vi "Test Parse State from Frame Name.vi"(8 "error in (no error)":errorcluster) -> (0 "error out":errorcluster)   [LabVIEW 2013, in "TEST JKI State Machine API.lvlib"]
uses:
  TEST JKI State Machine API.lvlib
  <vilib>/addons/_JKI Toolkits/Caraya/classes/Assert/Assert.lvclass
  <vilib>/addons/_JKI Toolkits/Caraya/classes/Test/Test.lvclass
  source/JKI SM/JKI SM.lvclass
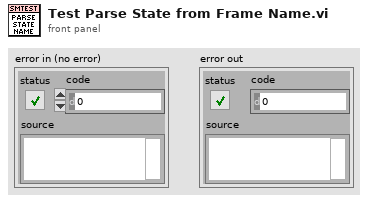
[diagram p1: front panel]
types:
  T1 = cluster{"Frame Name":string, "Exp'd Category":string, "Exp'd State":string, "Comment":string}[]
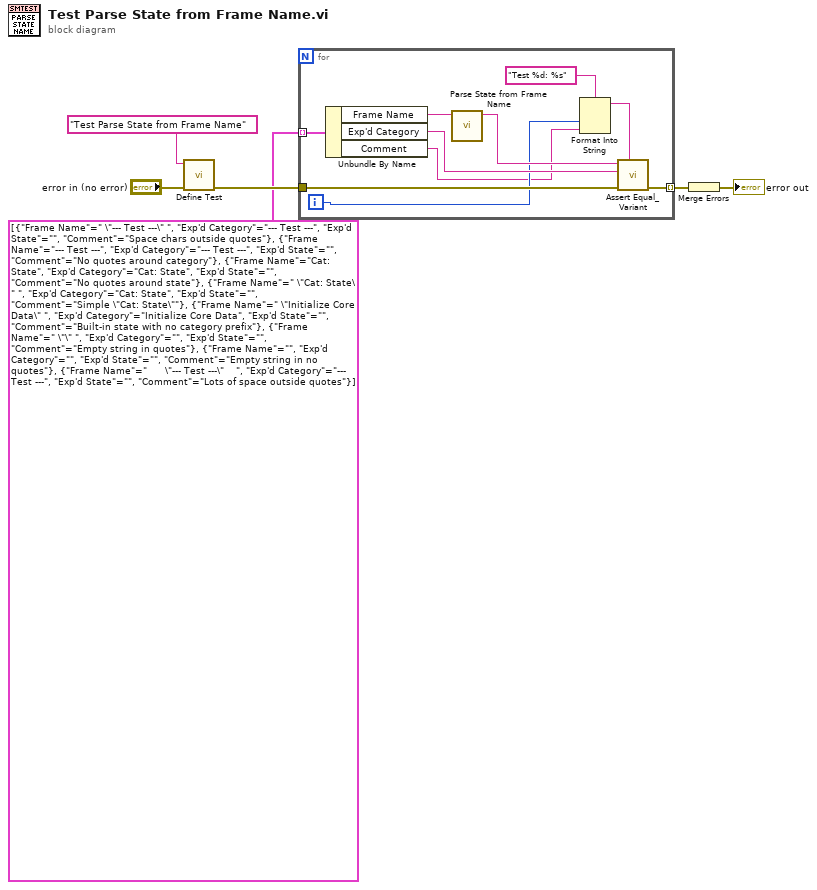
[diagram p0: block diagram]
diagram:
  n1 = call <vilib>:"Define Test.vi"("error in (no error)"="error in (no error)", "Label (VI Title)"="Test Parse State from Frame Name") -> ("error out"=w3:errorcluster)  [unwired: 9 in]
  n2 = for {
    tunnel: [w16] -> w4 mode=indexing
    tunnel: w3 -> [w15]
    tunnel: T1 [{"Frame Name"=" \"--- Test ---\" ", "Exp'd Category"="--- Test ---", "Exp'd State"="", "Comment"="Space chars outside quotes"}, {"Frame Name"="--- Test ---", "Exp'd Category"="--- Test ---", "Exp'd State"="", "Comment"="No quotes around category"}, {"Frame Name"="Cat: State", "Exp'd Category"="Cat: State", "Exp'd State"="", "Comment"="No quotes around state"}, {"Frame Name"=" \"Cat: State\" ", "Exp'd Category"="Cat: State", "Exp'd State"="", "Comment"="Simple \"Cat: State\""}, {"Frame Name"=" \"Initialize Core Data\" ", "Exp'd Category"="Initialize Core Data", "Exp'd State"="", "Comment"="Built-in state with no category prefix"}, {"Frame Name"=" \"\" ", "Exp'd Category"="", "Exp'd State"="", "Comment"="Empty string in quotes"}, {"Frame Name"="", "Exp'd Category"="", "Exp'd State"="", "Comment"="Empty string in no quotes"}, {"Frame Name"="      \"--- Test ---\"    ", "Exp'd Category"="--- Test ---", "Exp'd State"="", "Comment"="Lots of space outside quotes"}] -> [w14] mode=indexing
    i -> [w9]
    n3 = Unbundle By Name(w14) -> ("Frame Name"=w10:string, "Exp'd Category"=w11:string, "Comment"=w8:string)
    n4 = call "Parse State from Frame Name.vi"("Frame Name"=w10) -> ("Category Name"=w13:string)  [unwired: 7 in, 3 out]
    n5 = Format Into String(format string="Test %d: %s", w9, w8) -> (resulting string=w7:string)  [unwired: 2 in, 1 out]
    n6 = call <vilib>:"Assert Equal_Variant.vi"("Label"=w7, "error in (no error)"=w15, "Y"=w11, "X"=w13) -> ("error out"=w16:errorcluster)  [unwired: 7 in]
  }
  n7 = Merge Errors(w4) -> (→"error out":errorcluster)
